vi "use popup graph.vi"() -> ()   [LabVIEW 2015]
panel:
  out "# of values":i32
  out "temperature":dbl(slide) scale=0.0..100.0
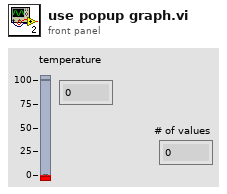
[diagram p1: front panel]
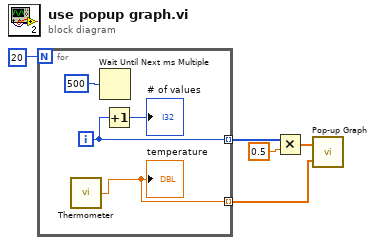
[diagram p0: block diagram]
diagram:
  n1 = for {
    N: 20 -> [_]
    tunnel: [w9] -> w4 mode=indexing
    tunnel: [w6] -> w1 mode=indexing
    i -> [w9]
    n2 = call "Thermometer.vi"() -> ("Thermometer"=w6:dbl)  [unwired: 1 in]
    "temperature" <- w6
    n3 = Wait Until Next ms Multiple(millisecond multiple=u32 500) -> ()  [unwired: 1 out]
    n4 = Increment(x=w9) -> (x+1=→"# of values":i32)
  }
  n5 = Multiply(x=w4, y=0.5) -> (x*y=w2:dbl[])
  n6 = call "Pop-up Graph.vi"("Y Array"=w1, "X Array"=w2) -> ()
